vi "LeadScrewFindHome (SubVI).vi"(8 "error in (no error)":errorcluster, 11 "miniOut in":T1) -> (0 "error out":errorcluster, 1 "LimitSW":bool, 2 "ENC Counter (deg/s)":dbl, 3 "miniOut out":T1)   [LabVIEW 2019]
uses:
  <vilib>/ReMiSYS/ReMiSYS_myRIO-mini/SubVI/SYS/miniRef.ctl
  <vilib>/Platform/TimedLoop/XDataNode/timing_clust.ctl
  <vilib>/Platform/TimedLoop/XDataNode/nitl_modes.ctl
  <vilib>/Platform/TimedLoop/XDataNode/wakeup.ctl
  <vilib>/platform/TimedLoop/XDataNode/XDataNode.xnode
  <vilib>/Platform/TimedLoop/XDataNode/XDNodeRunTimeDep.lvlib
panel:
  out "ENC Counter (deg/s) 2":dbl
  out "LimitSW 2":bool
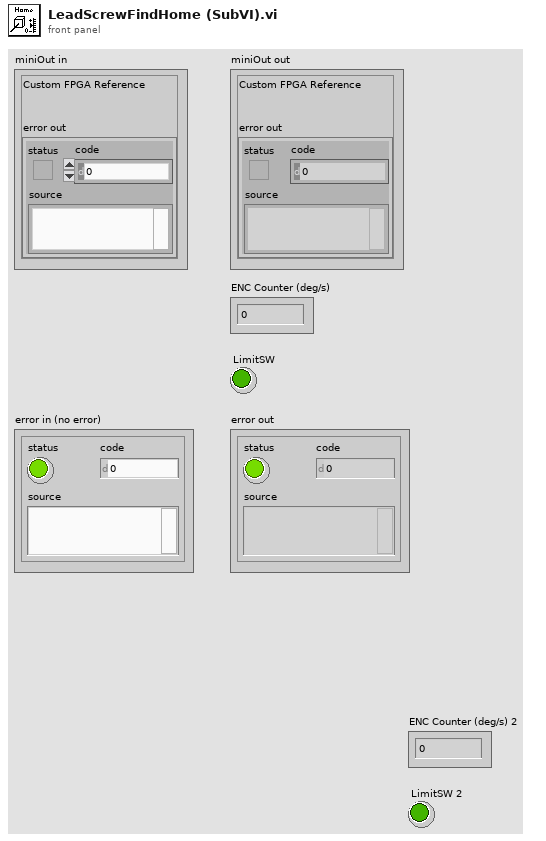
[diagram p1: front panel]
types:
  T1 = typedef "miniRef.ctl" = cluster{"Custom FPGA Reference":refnum<k20>, "error out":errorcluster}
  T2 = typedef "XDNodeRunTimeDep.lvlib/timing_clust.ctl" = cluster{"Expected End [f-1]":u64, "Actual End [f-1]":u64, "Finished Late? [f-1]":bool, "Expected End [i-1]":u64, "Actual End [i-1]":u64, "Finished Late? [i-1]":bool, "Expected Start [i]":u64, "Actual Start [i]":u64, "Expected Start [f]":u64, "Actual Start [f]":u64, "Source Name":string, "Structure Name":string, "Period":i64, "Deadline":i64, "Offset":i64, "Start":i64, "Priority":i32, "Timeout":i32, "Mode":T3, "Wakeup Reason":T4, "Error":errorcluster, "Source Type":string, "Secondary Source Type":string, "Global End Time":u64, "Global Start Time":u64, "Frame Duration":u64, "Iteration Duration":u64, "Assigned CPU":i32, "I/O Scan Engine Mode":u32}
  T3 = typedef "XDNodeRunTimeDep.lvlib/nitl_modes.ctl" = enum32{"No Change", "Process missed periods, maintain original phase", "Discard missed periods, maintain original phase", "Process missed periods, ignore original phase", "Discard missed periods, ignore original phase"}
  T4 = typedef "XDNodeRunTimeDep.lvlib/wakeup.ctl" = enum32{"Normal", "Aborted", "Asynchronous wakeup", "Timing source error", "Timed loop error", "Timeout"}
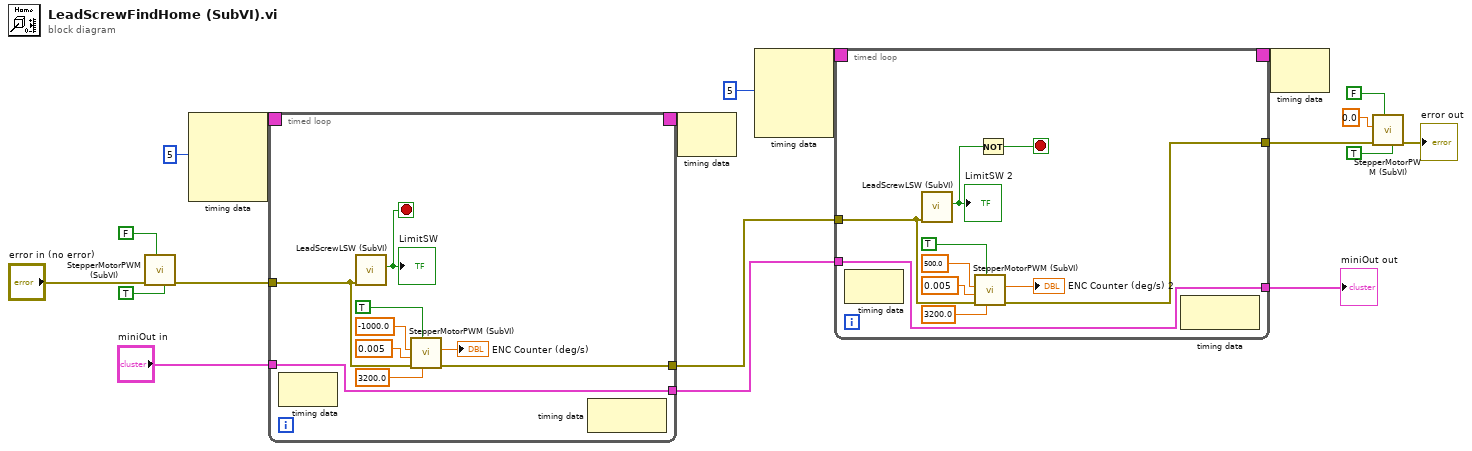
[diagram p0: block diagram]
diagram:
  n1 = call "StepperMotorPWM (SubVI).vi"("Reset"=TRUE, "EN"=FALSE, "error in (no error)"="error in (no error)") -> ("error out (no error)"=w3:errorcluster)  [unwired: 7 in, 1 out]
  n2 = node-c288(i64 5 ("Period")) -> (w19:T2)  [unwired: 3 in]
  n3 = timed-loop {
    timing: w19 -> [_]
    timing-out: [_] -> w18
    tunnel: [w28] -> w9
    tunnel: w3 -> [w22]
    tunnel: [w24] -> w11
    tunnel: "miniOut in" -> [w24]
    stop <- w20 stop-if-true
    n4 = node-c288() -> ()  [unwired: 1 in, 1 out]
    n5 = call "LeadScrewLSW (SubVI).vi"("error in (no error)"=w22) -> ("LeadScrewLimitSW"=w20:bool)  [unwired: 9 in, 1 out]
    "LimitSW" <- w20
    n6 = call "StepperMotorPWM (SubVI).vi"("steps/rev"=3200.0, "EN"=TRUE, "error in (no error)"=w22, "LoopTime"=0.005, "Speed (deg/s) [L,R]"=-1000.0) -> ("error out (no error)"=w28:errorcluster, "DegreeCounter"=→"ENC Counter (deg/s)":dbl)  [unwired: 5 in]
    n7 = node-c288() -> ()  [unwired: 1 in, 1 out]
  }
  n8 = node-c288(w18) -> ()  [unwired: 1 out]
  n9 = node-c288(i64 5 ("Period")) -> (w13:T2)  [unwired: 3 in]
  n10 = timed-loop {
    timing: w13 -> [_]
    timing-out: [_] -> w12
    tunnel: w9 -> [w36]
    tunnel: [w33] -> w7
    tunnel: w11 -> [w33]
    tunnel: [w31] -> w8
    stop <- w32 stop-if-true
    n11 = node-c288() -> ()  [unwired: 1 in, 1 out]
    n12 = call "LeadScrewLSW (SubVI).vi"("error in (no error)"=w36) -> ("LeadScrewLimitSW"=w34:bool)  [unwired: 9 in, 1 out]
    "LimitSW 2" <- w34
    n13 = call "StepperMotorPWM (SubVI).vi"("steps/rev"=3200.0, "EN"=TRUE, "error in (no error)"=w36, "LoopTime"=0.005, "Speed (deg/s) [L,R]"=500.0) -> ("error out (no error)"=w31:errorcluster, "DegreeCounter"=→"ENC Counter (deg/s) 2":dbl)  [unwired: 5 in]
    n14 = Not(x=w34) -> (.not. x?=w32:bool)
    n15 = node-c288() -> ()  [unwired: 1 in, 1 out]
  }
  "miniOut out" <- w7
  n16 = node-c288(w12) -> ()  [unwired: 1 out]
  n17 = call "StepperMotorPWM (SubVI).vi"("Reset"=TRUE, "EN"=FALSE ("EN [L,R]"), "error in (no error)"=w8, "Speed (deg/s) [L,R]"=0.0) -> ("error out (no error)"=→"error out":errorcluster)  [unwired: 6 in, 1 out]
